vi "start listening.vi"(8 "error in":errorcluster, 11 "TCP server in":refnum<class "TCP server.lvclass">) -> (0 "error out":errorcluster, 3 "TCP server out":refnum<class "TCP server.lvclass">)   [LabVIEW 2015, in "TCP server.lvclass"]
uses:
  TCP server.lvclass
  server/connection server.lvclass/connection server.ctl
  TCP server.lvclass/TCP server.ctl
  server/connection server.lvclass
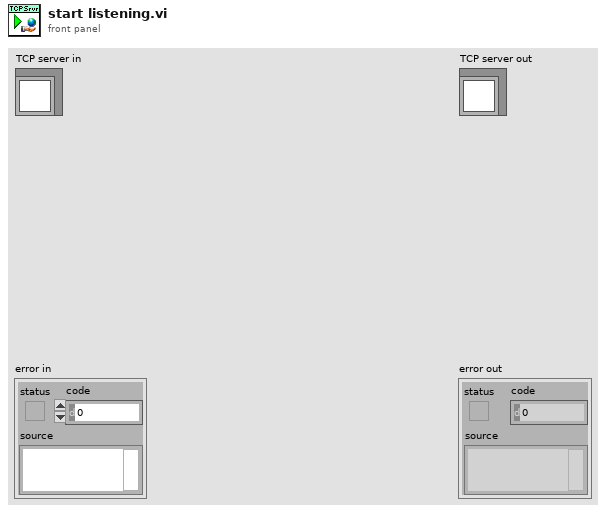
[diagram p1: front panel]
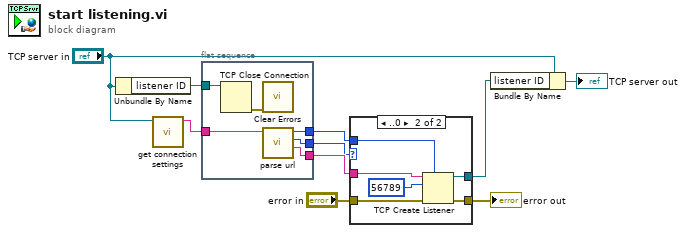
[diagram p0: block diagram]
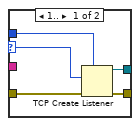
[diagram p2: hidden frame]
diagram:
  n1 = Unbundle By Name("TCP server in") -> ("listener ID"=w3:refnum<k5>)
  n2 = call "get connection settings.vi"("connection server in"="TCP server in") -> ("connection string"=w1:string)  [unwired: 9 in, 1 out]
  n3 = flat-sequence {
    tunnel: [w16] -> w10
    tunnel: [w15] -> w9
    tunnel: [w14] -> w8
    tunnel: w3 -> [w13]
    tunnel: w1 -> [w11]
    frame #0 {
      n4 = TCP Close Connection(connection ID=w13) -> (error out=w12:errorcluster)  [unwired: 2 in, 1 out]
      n5 = call <vilib>:"Clear Errors.vi"("error in (no error)"=w12) -> ()  [unwired: 5 in, 2 out]
      n6 = call "parse url.vi"("connection string in"=w11) -> ("service"=w15:string, "port"=w14:u16, "net address"=w16:u32)  [unwired: 8 in]
    }
  }
  n7 = case shown="..0" w8 {
    selector: w8 -> [w20 _]
    tunnel: w10 -> [w21 w27]
    tunnel: w9 -> [_ w26]
    tunnel: [w19 w24] -> w7
    tunnel: [w18 w23] -> w5
    tunnel: "error in" -> [w17 w22]
    frame 1.. {
      n8 = TCP Create Listener(7:w21, 8:w17, 10:w20) -> (0:w19:errorcluster, 3:w18:refnum<k5>)  [unwired: 2 in, 1 out]
    }
    frame ..0 {
      n9 = TCP Create Listener(7:w27, 8:w22, 10:u16 56789 ("port"), 11:w26) -> (0:w24:errorcluster, 3:w23:refnum<k5>)  [unwired: 1 in, 1 out]
    }
  }
  "error out" <- w7
  n10 = Bundle By Name(cluster="TCP server in", "listener ID"=w5) -> (→"TCP server out":refnum<class "TCP server.lvclass">)
